vi "ACQ.vi"(8 "errorIn":errorcluster, 11 "xmlFilePath":path) -> (0 "error out":errorcluster caption="errorOut", 3 "ACQ":T1)   [LabVIEW 2017]
uses:
  models/ACQ.ctl
  models/Header.ctl
  models/ACQ_channel.ctl
  <vilib>/xml/Load XML File.vi
  <vilib>/xml/NI_XML.lvlib
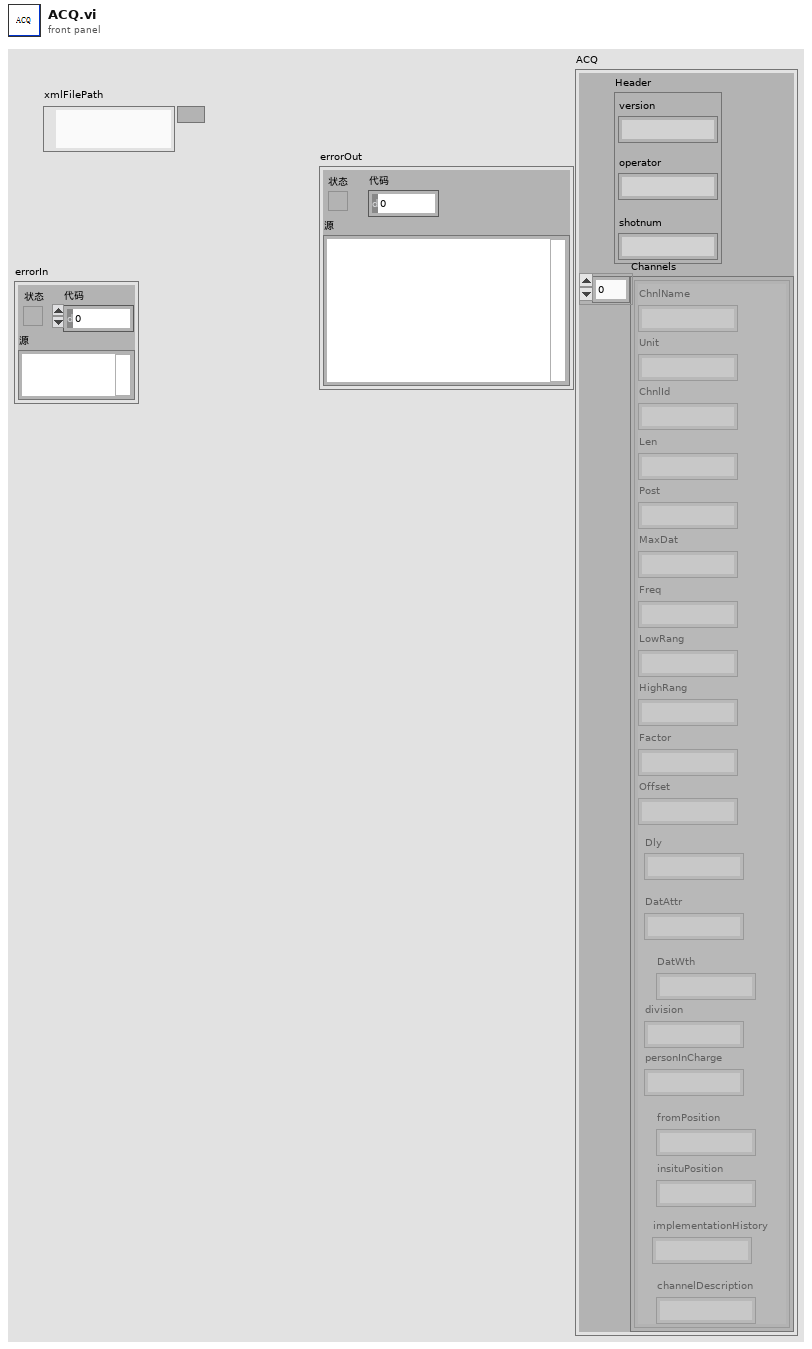
[diagram p1: front panel]
types:
  T1 = typedef "ACQ.ctl" = cluster{"Header":T2, "Channels":T3[]}
  T2 = typedef "Header.ctl" = cluster{"version":string, "operator":string, "shotnum":string}
  T3 = typedef "ACQ_channel.ctl" = cluster{"ChnlName":string, "Unit":string, "ChnlId":string, "Len":string, "Post":string, "MaxDat":string, "Freq":string, "LowRang":string, "HighRang":string, "Factor":string, "Offset":string, "Dly":string, "DatAttr":string, "DatWth":string, "division":string, "personInCharge":string, "fromPosition":string, "insituPosition":string, "implementationHistory":string, "channelDescription":string}
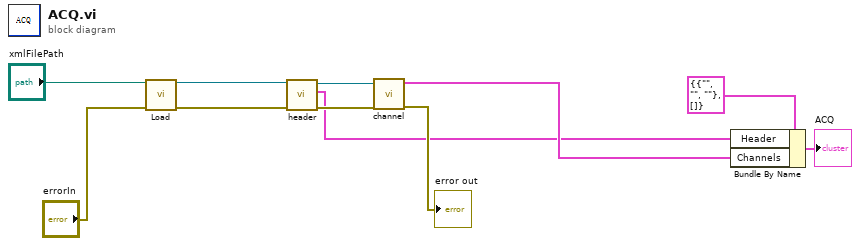
[diagram p0: block diagram]
diagram:
  n1 = call-poly <vilib>:"Load.vi"("path to XML document"="xmlFilePath", "error in (no error)"="errorIn") -> ("DOM document out"=w8:refnum<k20>, "error out"=w5:errorcluster)  [unwired: 11 in, 1 out]
  n2 = call "header.vi"("errorIn"=w5, "xmlRef"=w8) -> ("errorOut"=w10:errorcluster, "header"=w2:T2, "xmlRef"=w11:refnum<k20>)  [unwired: 7 in]
  n3 = call "channel.vi"("error in"=w10, "xmlRef"=w11) -> ("error out"=→"error out":errorcluster, "channels"=w3:T3[])  [unwired: 8 in]
  n4 = Bundle By Name(cluster=T1 {"Header"={"version"="", "operator"="", "shotnum"=""}, "Channels"=[]} ("输入簇"), "Header"=w2, "Channels"=w3) -> (→"ACQ":T1)
